vi "Initialise.vi"(4 "error IO":errorcluster, 5 "X,Y,Z values":T1={"mm Xmin "=0.0, "mm Xmax "=100.0, " mm Ymin "=0.0, "mm Ymax "=267.9, " mm Zmin"=0.0, "mm Zmax "=108.0, "Schritte oder mm Umin (0)"=0.0, "Schritte oder mm Umax (0)"=0.0, "Schritte oder mm Cmin (0)"=0.0, "Schritte oder mm Cmax (0)"=0.0, "Schritte oder mm Amin (0)"=0.0, "Schritte oder mm Amax (0)"=0.0, "Schritte oder mm Bmin (0)"=0.0, "Schritte oder mm Bmax (0)"=0.0}, 6 "String":string, 7 "Port for KOSY3":refnum<visa-resource-name>) -> (0 "Fehler (Ausgang)":errorcluster, 1 "Cordinates of the  KOSY3 Platform":T2 {"Schritte B" format="%#.4g"; "Schritte A" format="%#.4g"; "Schritte C" format="%#.4g"; "Schritte U" format="%#.4g"; "Schritte Z" format="%#.4g"; "Schritte Y" format="%#.4g"; "Schritte X" format="%#.4g"}, 2 "String 2":string, 3 "VISA-Referenz (Ausgang)":refnum<visa-resource-name>)   [LabVIEW 2013]
panel:
  out "Speed":dbl(knob) scale=0.0..20.0
  out "Stopped":bool
  out "Moving":bool
  out "Status":string="Initialise"
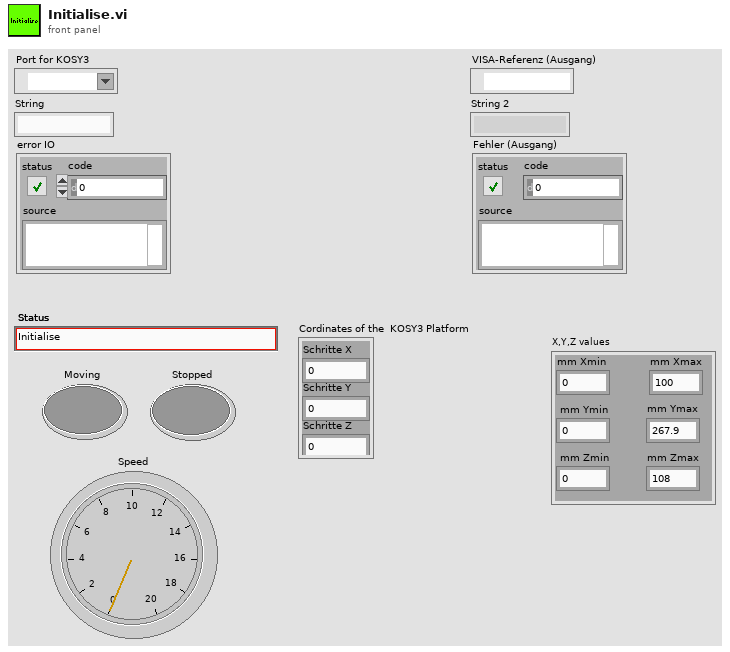
[diagram p1: front panel]
types:
  T1 = cluster{"mm Xmin ":sgl, "mm Xmax ":sgl, " mm Ymin ":sgl, "mm Ymax ":sgl, " mm Zmin":sgl, "mm Zmax ":sgl, "Schritte oder mm Umin (0)":sgl, "Schritte oder mm Umax (0)":sgl, "Schritte oder mm Cmin (0)":sgl, "Schritte oder mm Cmax (0)":sgl, "Schritte oder mm Amin (0)":sgl, "Schritte oder mm Amax (0)":sgl, "Schritte oder mm Bmin (0)":sgl, "Schritte oder mm Bmax (0)":sgl}
  T2 = cluster{"Schritte X":sgl, "Schritte Y":sgl, "Schritte Z":sgl, "Schritte U":sgl, "Schritte C":sgl, "Schritte A":sgl, "Schritte B":sgl}
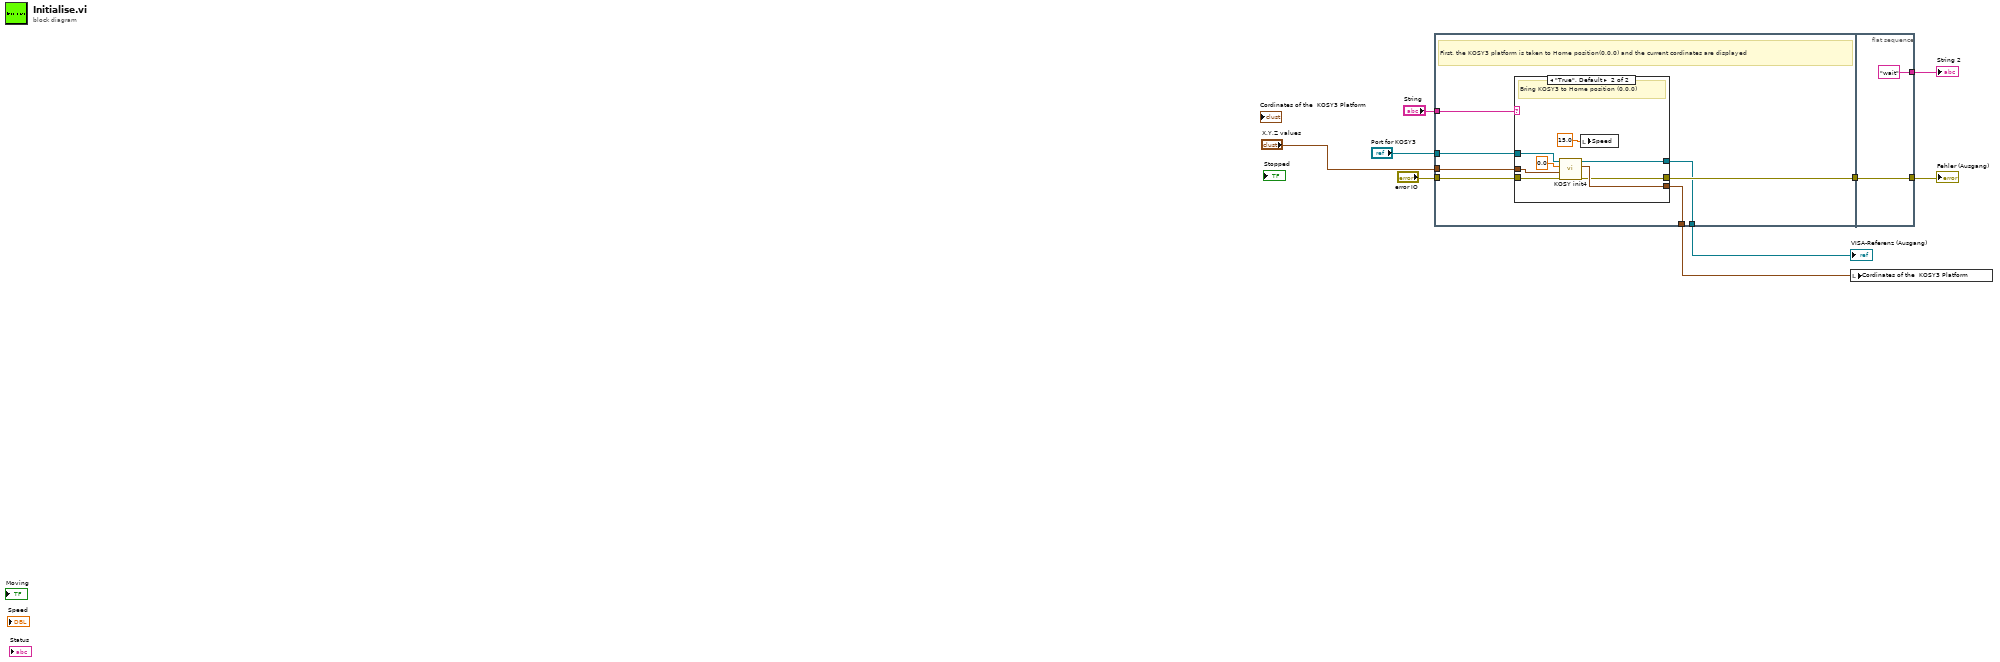
[diagram p0: block diagram]
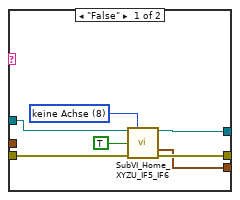
[diagram p2: hidden frame]
diagram:
  n1 = flat-sequence {
    tunnel: "error IO" -> [w16]
    tunnel: [w15] -> w9
    tunnel: "String" -> [w14]
    tunnel: "Port for KOSY3" -> [w13]
    tunnel: [w12] -> w5
    tunnel: [w11] -> w2
    tunnel: "X,Y,Z values" -> [w10]
    tunnel: w9 -> [w33]
    tunnel: [w33] -> w3
    tunnel: ["wait"] -> w4
    frame #0 {
      # "First, the KOSY3 platform is taken to Home position(0,0,0) and the current cordinates are displayed"
      n2 = case shown="\"True\", Default" w14 {
        tunnel: [w21 w28] -> w15
        tunnel: w16 -> [w20 w30]
        tunnel: [w19 w29] -> w11
        tunnel: w10 -> [_ w27]
        tunnel: w13 -> [w18 w25]
        tunnel: [w17 w24] -> w12
        frame "False" {
          w22 = u16 8 items=["X-Achse", "Y-Achse", "Z-Achse", "X- und Y-Achse", "X- und Z-Achse", "Y- und Z-Achse", "X, Y und Z-Achse", "U-Achse", "keine Achse"] ("Beteiligte Achsen (X,Y,Z,U)")
          n3 = call "SubVI_Home_XYZU_IF5_IF6.vi"("VISA resource name in"=w18, "Beteiligte Achsen (X,Y,Z,U)"=w22, "IF5=F/IF6=T\n(IF6=T) in"=TRUE ("IF5=F/IF6=T\n(IF6=T) in"), "error in"=w20) -> ("VISA resource name out"=w17:refnum<visa-resource-name>, "Koordinaten IF6"=w19:T2, "error out"=w21:errorcluster)  [unwired: 4 in, 5 out]
        }
        frame "True", Default {
          # "Bring KOSY3 to Home position (0,0,0)"
          n4 = call "KOSY init4.vi"("error in (no error)"=w30, "Bereiche IF6 X,Y,Z,U,C,A,B\n(X:0-310,Y:0-275,Z:0-108,U:0,C:0,A:0,B:0)"=w27, "Numerisch"=0.0, "VISA-Referenz (Eingang)"=w25) -> ("Fehler (Ausgang)"=w28:errorcluster, "Coordinates IF6"=w29:T2, "VISA-Referenz (Ausgang)"=w24:refnum<visa-resource-name>)  [unwired: 4 in, 1 out]
          n5 = local write "Speed"(15.0 ("Speed")) -> ()
        }
      }
    }
    frame #1 {
    }
  }
  n6 = local write "Cordinates of the  KOSY3 Platform"(w2) -> ()
  "VISA-Referenz (Ausgang)" <- w5
  "String 2" <- w4
  "Fehler (Ausgang)" <- w3
